vi "dem san pham vi.vi"() -> ()   [LabVIEW 2020]
uses:
  <vilib>/MakerHub/LINX/Public/Peripherals/Digital/Digital Read 1 Chan.vi
  <vilib>/MakerHub/LINX/Public/Peripherals/Digital/Digital Read N Chans.vi
  <vilib>/MakerHub/LINX/Private/Local IO/LinxDigitalRead.vi
  <vilib>/MakerHub/LINX/Public/Utilities/Check Channel.vi
  <vilib>/MakerHub/LINX/Public/Utilities/Open Serial.vi
  <vilib>/MakerHub/LINX/Private/Utilties/Generate Error.vi
  <vilib>/functionblocks/Counter/Count Up/Count Up.vi
  <vilib>/functionblocks/FB Core/FB Core.xnode
  <vilib>/MakerHub/LINX/LMH-LINX.lvlib
  <vilib>/functionblocks/NI_FunctionBlock Libraries.lvlib
panel:
  out "done":bool
  out "counter value":u32
  in  "reset":bool
  in  "preset value":u32=10
  in  "stop":bool
  in  "Serial Port":refnum<visa-resource-name>="N/A"
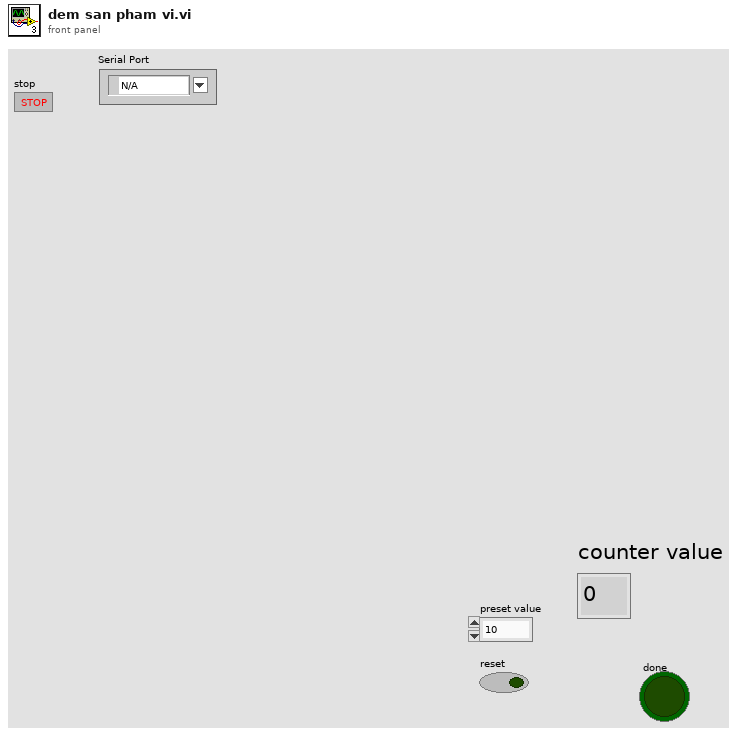
[diagram p1: front panel]
types:
  T1 = typedef "LMH-LINX.lvlib/LINX Ref.ctl" = cluster{"IO":T2, "Interface":T3, "LINX Device Config":T4}
  T2 = typedef "LMH-LINX.lvlib/Platform.ctl" = enum16{"Remote", "Local"}
  T3 = typedef "LMH-LINX.lvlib/Interface.ctl" = enum16{"Serial", "TCP"}
  T4 = typedef "LMH-LINX.lvlib/Device.lvlib/LINX Device Config.ctl" = cluster{"Interface":T3, "COM Port":refnum<visa-resource-name>, "TCP Configuration":T5, "Device Family":u8, "Device ID":u8, "Device Name":string, "TCP Ref":refnum<k5>, "Channels":T6}
  T5 = typedef "LMH-LINX.lvlib/Device.lvlib/TCP Config.ctl" = cluster{"IP Address":string, "Port":u16}
  T6 = typedef "LMH-LINX.lvlib/Channels.ctl" = cluster{"DI":u8[], "DO":u8[], "AI":u8[], "AO":u8[], "PWM":u8[], "QE":u8[], "UART":u8[], "I2C 2":u8[], "SPI":u8[], "CAN":u8[], "Servo":u8[], "AI Ref (V)":dbl, "AI Resolution (Bits)":u8, "AO Ref (V)":dbl, "AO Resolution (Bits)":u8}
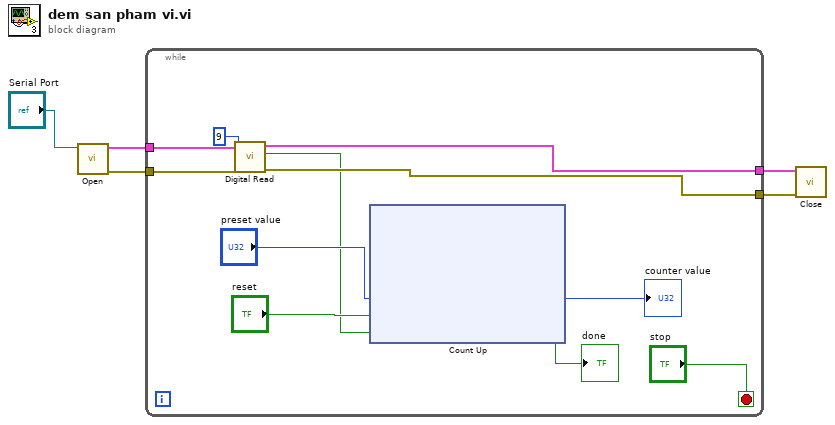
[diagram p0: block diagram]
diagram:
  n1 = call-poly <vilib>:"Open.vi"("Serial Port"="Serial Port") -> ("Error Out"=w3:errorcluster, "LINX Resource"=w5:T1)  [unwired: 8 in, 1 out]
  n2 = while {
    tunnel: w5 -> [w16]
    tunnel: [w15] -> w4
    tunnel: w3 -> [w14]
    tunnel: [w13] -> w2
    stop <- "stop" stop-if-true
    n3 = call-poly <vilib>:"Digital Read.vi"("Error In"=w14, "DI Channel"=u8 9, "LINX Resource"=w16) -> ("Error Out"=w13:errorcluster, "DI Value"=w8:bool, "LINX Resource"=w15:T1)  [unwired: 6 in]
    n4 = xnode "Count Up"("preset value"="preset value", "reset"="reset", "count up"=w8) -> ("counter value"=→"counter value":u32, "done"=→"done":bool)  [unwired: 1 in, 1 out]
  }
  n5 = call <vilib>:"Close.vi"("Error In"=w2, "LINX Resource"=w4) -> ()  [unwired: 9 in, 1 out]
